vi "getO3FolderContent.vi"(7 "LWRS":refnum<class "Web Request.lvclass">) -> ()   [LabVIEW 2014]
uses:
  <vilib>/wsapi/Web Request.lvclass
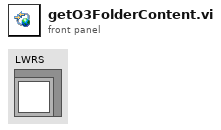
[diagram p1: front panel]
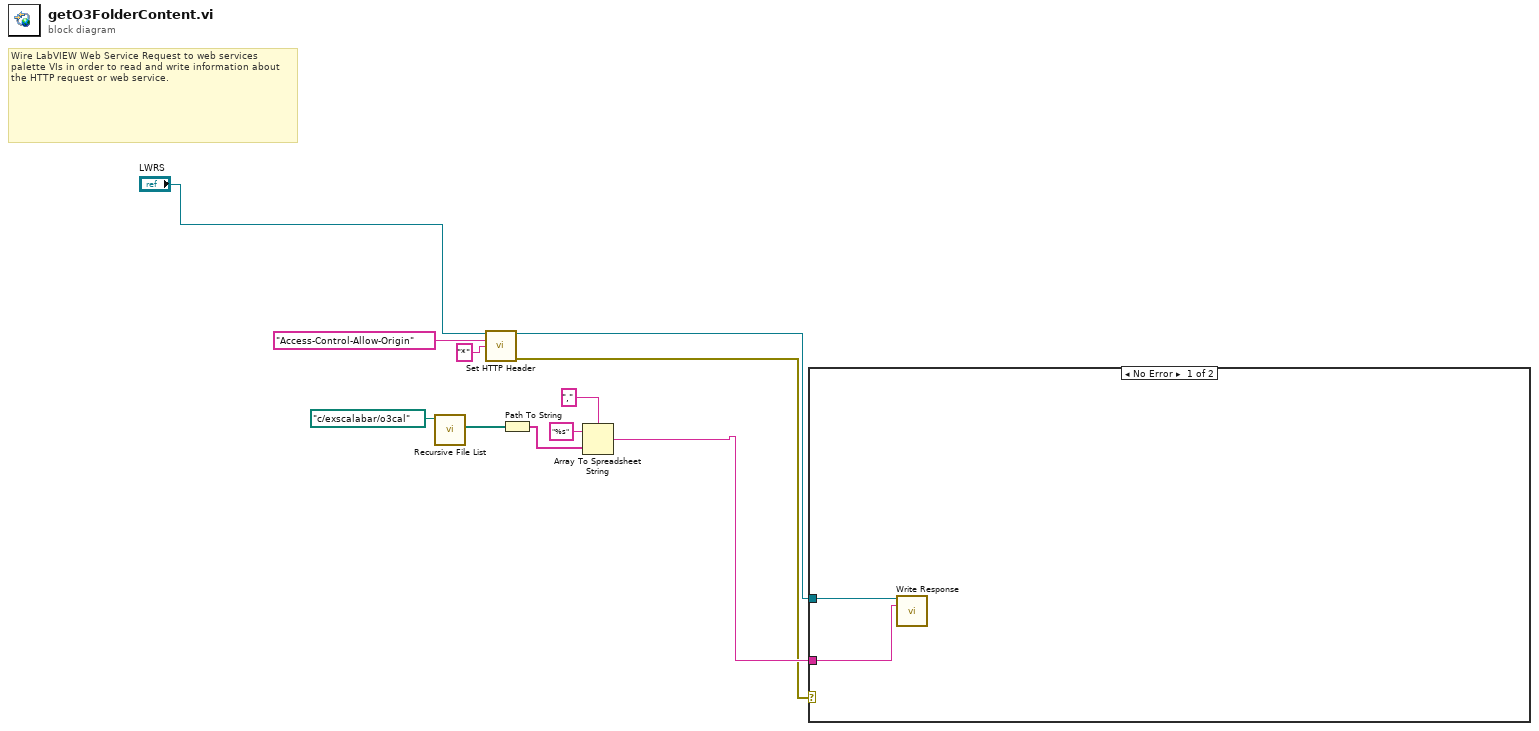
[diagram p0: block diagram]
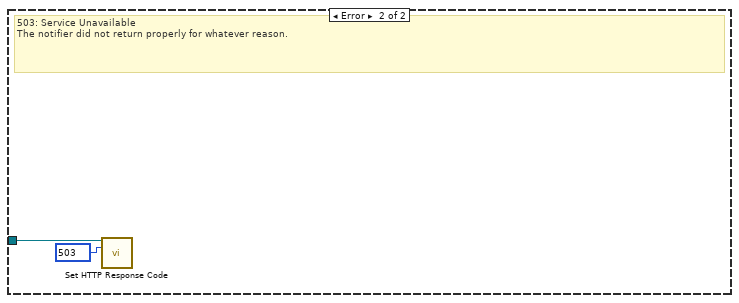
[diagram p2: hidden frame]
diagram:
  # "Wire LabVIEW Web Service Request to web services palette VIs in order to read and write information about the HTTP request or web service."
  n1 = call <vilib>:"Recursive File List.vi"("Folder Path"=path "c:/exscalabar/o3cal") -> ("All Files in Dir"=w7:path[])  [unwired: 6 in, 4 out]
  n2 = call <vilib>:"Set HTTP Header.vi"("LabVIEW Web Service Request"="LWRS", "header"="Access-Control-Allow-Origin", "header value"="*") -> ("LabVIEW Web Service Request out"=w3:refnum<class "Web Request.lvclass">, "error out"=w1:errorcluster)  [unwired: 11 in]
  n3 = Path To String(path=w7) -> (string=w6:string[])
  n4 = Array To Spreadsheet String(delimiter (Tab)=",", array=w6, 3:"%s" ("format string")) -> (spreadsheet string=w2:string)
  n5 = case shown="No Error" w1 {
    tunnel: w3 -> [w13 w15]
    tunnel: w2 -> [w12 _]
    frame No Error {
      n6 = call <vilib>:"Write Response.vi"("LabVIEW Web Service Request"=w13, "response string"=w12) -> ()  [unwired: 12 in, 2 out]
    }
    frame Error {
      w14 = 503 items=["100"=100, "101"=101, "200"=200, "201"=201, "202"=202, "203"=203, "204"=204, "205"=205, "206"=206, "300"=300, "301"=301, "302"=302, "303"=303, "304"=304, "305"=305, "306"=306, "307"=307, "400"=400, "401"=401, "402"=402, "403"=403, "404"=404, "405"=405, "406"=406, "407"=407, "408"=408, "409"=409, "410"=410, "411"=411, "412"=412, "413"=413, "414"=414, "415"=415, "416"=416, "417"=417, "500"=500, "501"=501, "502"=502, "503"=503, "504"=504, "505"=505] ("response code (200)")
      # "503: Service Unavailable\nThe notifier did not return properly for whatever reason."
      n7 = call <vilib>:"Set HTTP Response Code.vi"("LabVIEW Web Service Request"=w15, "response code (200)"=w14) -> ()  [unwired: 12 in, 2 out]
    }
  }
